vi "Simulation - Tank Level RT demo2.vi"() -> ()   [LabVIEW 2025]
doc: "This example demonstrates a process simulation for a tank level. The process has added noise, valve deadband, lag, and deadtime. A level controller adjusts the inflow to a tank. An on/off valve serves as a drain that you can click on to operate. This s-valve represents a change in the process loading. You also can switch this VI from automatic control to manual control."
uses:
  <vilib>/addons/control/pid/NI_PID_pid.lvlib
  <vilib>/addons/control/pid/pid.llb/PID Advanced (DBL).vi
panel:
  in  "Physical Model":bool=TRUE
  in  "Tab Control":enum32{"Introduction", "Operation"}(tab)=enum."Operation"
  out "Flow sensor":bool
  in  "HV-101":bool
  out "tank level":dbl(slide) scale=0.0..100.0 scale format="%#.2g"
  out "Valve":bool
  in  "LCV-101":dbl(knob) scale=0.0..100.0
  in  "Auto":bool=TRUE
  out "Process Chart":T1(graph)={"initial PV"=18.934717983735947, "SP(%)"=34.59119496855346, "output"=100.0}
  in  "Setpoint":dbl(slide)=50.0 scale=0.0..100.0
  in  "PID parameters (LIC 101)":T2={"Kc"=10.0, "Ti (min)"=0.05, "Td (min)"=0.0} {"Td (min)" format="%#.6f"; "Ti (min)" format="%#.4f"; "Kc" format="%#.4f"}
  in  "Stop":bool
  # "Tank Level Control"
  # "Overview: This example demonstrates a process simulation for a tank level.  The process has added noise, valve deadband, lag, and deadtime.  A level controller adjusts the inflow to a tank.  An on/off valve serves as a drain that you can click on to operate.  This s-valve represents a change in the process loading.  You also can switch this VI from automatic control to manual control.\nInstructions:\n1. Run the VI.\n2. Verify the PID controller in closed-loop to track the setpoint.\n3. Change the setpoint to another value and verify the controller tracking the new setpoint.\n4. Apply a disturbance to the system by switching the valve HV 102 (click on the valve symbol). You will see the controller recovering fro the change.\n5. Change PID gains and see if you can improve its performance without going unstable.\n6. Switch to manual mode and see if you can control the level by changing the Valve LVC 101.\n7. Click Stop to stop the VI."
  # "ISA Symbology: The diagram uses the ISA Symbology used for control"
  # "Loop 101"
  # "Level Controller at the control room"
  # "Level Transmitter on the field"
  # "Level Control Valve on the field"
  # "Hand Control Valve on the field"
  # "HV"
  # "102"
  # "LCV"
  # "101"
  # "LIC"
  # "101"
  # "LT"
  # "101"
  # "Slow Leak"
  # "Click to operate"
  # "HV"
  # "102"
  # "LCV"
  # "101"
  # "LIC"
  # "101"
  # "LT"
  # "101"
  # "Manual"
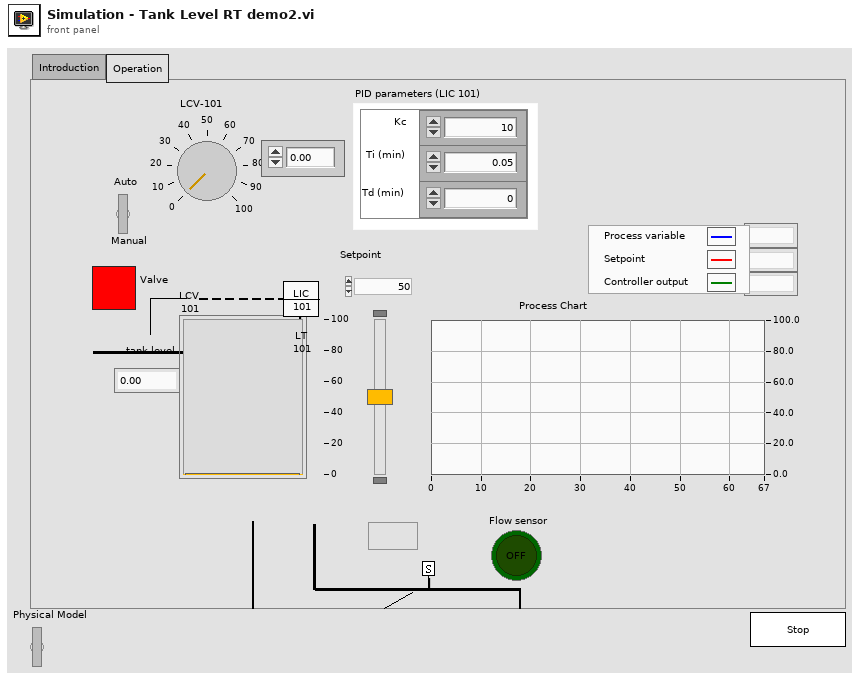
[diagram p1: front panel]
types:
  T1 = cluster{"initial PV":dbl, "SP(%)":dbl, "output":dbl}
  T2 = cluster{"Kc":dbl, "Ti (min)":dbl, "Td (min)":dbl}
  T3 = cluster{"static gain":dbl, "lag (s)":dbl, "deadtime (s)":dbl, "load":dbl, "deadband":dbl, "sensor noise":dbl, "initial PV":dbl, "plant noise":dbl}
  T4 = cluster{"Plant Output":dbl, "Setpoint":dbl, "output":dbl}
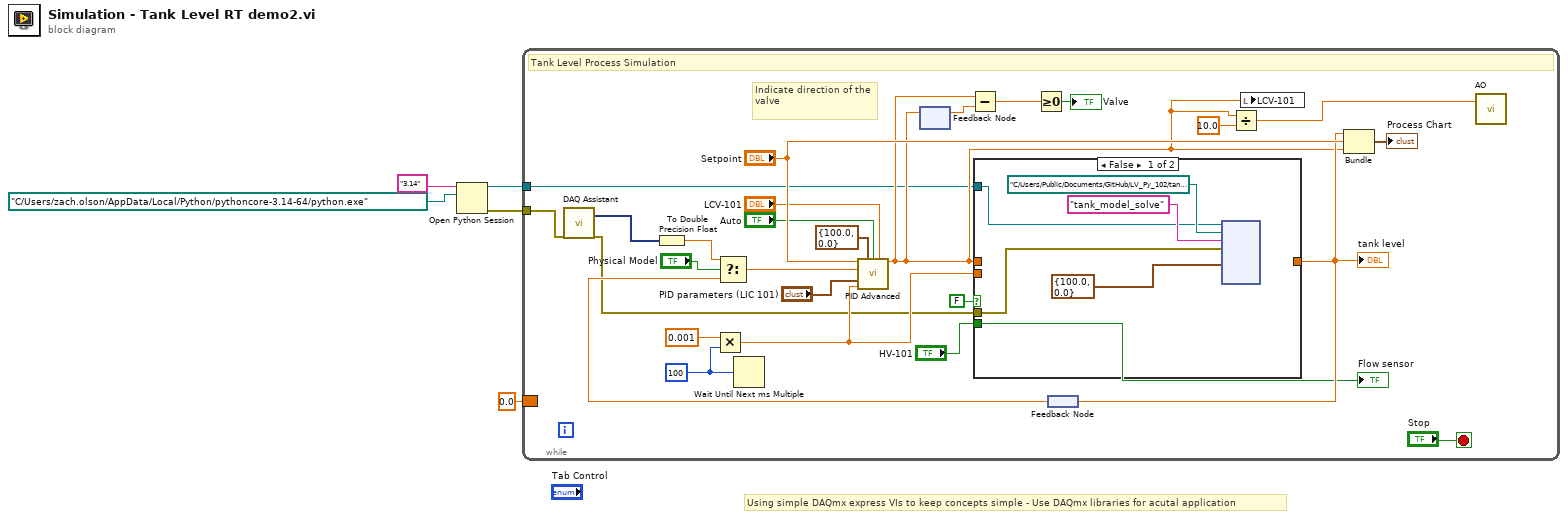
[diagram p0: block diagram]
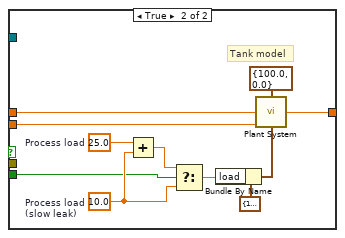
[diagram p2: hidden frame]
diagram:
  # "Using simple DAQmx express VIs to keep concepts simple - Use DAQmx libraries for acutal application"
  n1 = Open Python Session(python version="3.14" ("Python version"), python path=path "C:/Users/zach.olson/AppData/Local/Python/pythoncore-3.14-64/python.exe" ("Python path")) -> (session out=w2:refnum<k35>, error out=w1:errorcluster)  [unwired: 1 in]
  n2 = while {
    border: 0.0 ("Plant Output") -> [_]
    tunnel: w2 -> [w9]
    tunnel: w1 -> [w8]
    stop <- "Stop" stop-if-true
    w24 = u32 100
    # "Indicate direction of the valve"
    # "Tank Level Process Simulation"
    n3 = call "DAQ Assistant"("error in"=w8) -> ("data"=w10:dynamicdata, "error out"=w7:errorcluster)  [unwired: 16 in, 1 out]
    n4 = To Double Precision Float(number=w10) -> (double precision float=w11:dbl)
    n5 = Multiply(x=0.001, y=w24) -> (x*y=w23:dbl)
    n6 = Wait Until Next ms Multiple(millisecond multiple=w24) -> ()  [unwired: 1 out]
    n7 = feedback #1() -> (w21:dbl)  [unwired: 1 in]
    n8 = feedback #2() -> (w13:dbl)
    n9 = Select(t=w11, s="Physical Model", f=w13) -> (s? t:f=w14:dbl)
    n10 = call-poly <vilib>:"PID Advanced.vi"("setpoint"="Setpoint", "output range"=cluster{"output high":dbl, "output low":dbl} {"output high"=100.0, "output low"=0.0}, "auto? (T)"="Auto", "manual control"="LCV-101", "process variable"=w14, "PID gains"="PID parameters (LIC 101)", "dt (s)"=w23) -> ("output"=w17:dbl)  [unwired: 7 in, 1 out]
    n11 = feedback-in #1(w17) -> ()
    n12 = Subtract(x=w17, y=w21) -> (x-y=w20:dbl)
    n13 = case shown="False" FALSE {
      tunnel: w23 -> [_ w44]
      tunnel: [_ w43] -> w22
      tunnel: "HV-101" -> [_ w39]
      tunnel: w17 -> [_ w38]
      tunnel: w9 -> [w35 _]
      tunnel: w7 -> [w34 _]
      frame False {
        n14 = node(w35, path "C:/Users/Public/Documents/GitHub/LV_Py_102/tank.py" ("module path"), "tank_model_solve" ("function name"), w34, cluster{"output high":dbl, "output low":dbl} {"output high"=100.0, "output low"=0.0} ("output saturation range")) -> ()  [unwired: 7 in, 4 out]
      }
      frame True {
        w42 = 10.0  # Process load (slow leak)
        w41 = 25.0  # Process load
        # "Tank model"
        n15 = Add(x=w41, y=w42) -> (x+y=w40:dbl)
        n16 = Select(t=w40, s=w39, f=w42) -> (s? t:f=w46:dbl)
        n17 = Bundle By Name(cluster=T3 {"static gain"=1.5, "lag (s)"=18.0, "deadtime (s)"=1.0, "load"=0.0, "deadband"=1.0, "sensor noise"=0.0, "initial PV"=0.0, "plant noise"=5.0} ("process parameters"), "load"=w46) -> (w45:T3)
        n18 = call "Plant System.vi"("output saturation range"=cluster{"output high":dbl, "output low":dbl} {"output high"=100.0, "output low"=0.0}, "Plant Input"=w38, "dt (s)"=w44, "process parameters"=w45) -> ("Plant Output"=w43:dbl)  [unwired: 11 in]
      }
    }
    "tank level" <- w22
    n19 = Greater Or Equal To 0?(x=w20) -> (x >= 0?=→"Valve":bool)
    n20 = feedback-in #2(w22) -> ()
    n21 = Divide(x=w17, y=10.0) -> (x/y=w15:dbl)
    n22 = local write "LCV-101"(w17) -> ()
    n23 = Bundle("Plant Output"=w22, "Setpoint"="Setpoint", "output"=w17) -> (→"Process Chart":T4)  [unwired: 1 in]
    n24 = call "AO"("data"=w15) -> ()  [unwired: 17 in, 2 out]
    "Flow sensor" <- "HV-101"
  }
